vi "GetBoolFromNode(viaStringNodePath).vi"(2 "Path":string, 3 "error in":errorcluster, 5 "Tree DVR in":refnum<data-value>) -> (0 "error out":errorcluster, 1 "Bool Out":bool)   [LabVIEW 2014]
uses:
  <vilib>/MDSplus/Classes/Tree_Class/Tree.lvclass
  <vilib>/MDSplus/Library/MDSplus.lvlib
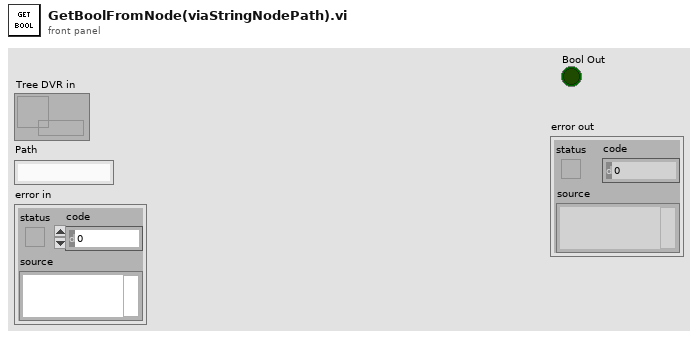
[diagram p1: front panel]
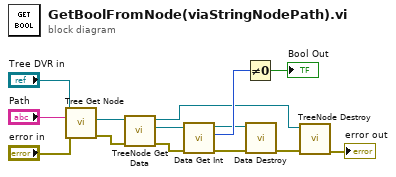
[diagram p0: block diagram]
diagram:
  n1 = call <vilib>:"Tree Get Node.vi"("error in (no error)"="error in", "Path"="Path", "Tree DVR in"="Tree DVR in") -> ("error out"=w13:errorcluster, "Node out"=w14:refnum<data-value>)  [unwired: 6 in, 1 out]
  n2 = call <vilib>:"TreeNode Get Data.vi"("error in (no error)"=w13, "TreeNode DVR in"=w14) -> ("error out"=w12:errorcluster, "Data out"=w11:refnum<data-value>, "TreeNode DVR out"=w3:refnum<data-value>)  [unwired: 7 in]
  n3 = call <vilib>:"Data Get Int.vi"("error in (no error)"=w12, "Data DVR in"=w11) -> ("error out"=w5:errorcluster, "I32 out"=w8:i32, "Data DVR out"=w6:refnum<data-value>)  [unwired: 7 in]
  n4 = Not Equal To 0?(x=w8) -> (x != 0?=→"Bool Out":bool)
  n5 = call <vilib>:"Data Destroy.vi"("error in (no error)"=w5, "Data DVR in"=w6) -> ("error out"=w4:errorcluster)  [unwired: 9 in]
  n6 = call <vilib>:"TreeNode Destroy.vi"("error in (no error)"=w4, "TreeNode DVR in"=w3) -> ("error out"=→"error out":errorcluster)  [unwired: 9 in]
